vi "LNLS Control Encode FOFBC.vi"(8 "error in (no error)":errorcluster, 11 "LNLS Control FOFB Configuration":T1) -> (0 "error out":errorcluster, 2 "command body":string)   [LabVIEW 2011, in "LNLS Control VIs.lvlib"]
uses:
  LNLS Control VIs.lvlib
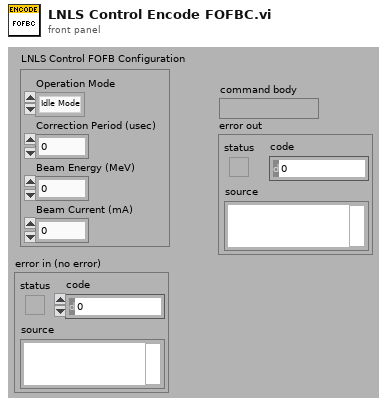
[diagram p1: front panel]
types:
  T1 = cluster{"Operation Mode":enum16{"Idle Mode", "Error Mode", "Manual Mode", "FOFB Mode", "RMM Mode"}, "Correction Period (usec)":i32, "Beam Energy (MeV)":sgl, "Beam Current (mA)":sgl}
  T2 = enum16{"big-endian, network order", "native, host order", "little-endian"}
  T3 = enum16{"Idle Mode", "Error Mode", "Manual Mode", "FOFB Mode", "RMM Mode"}
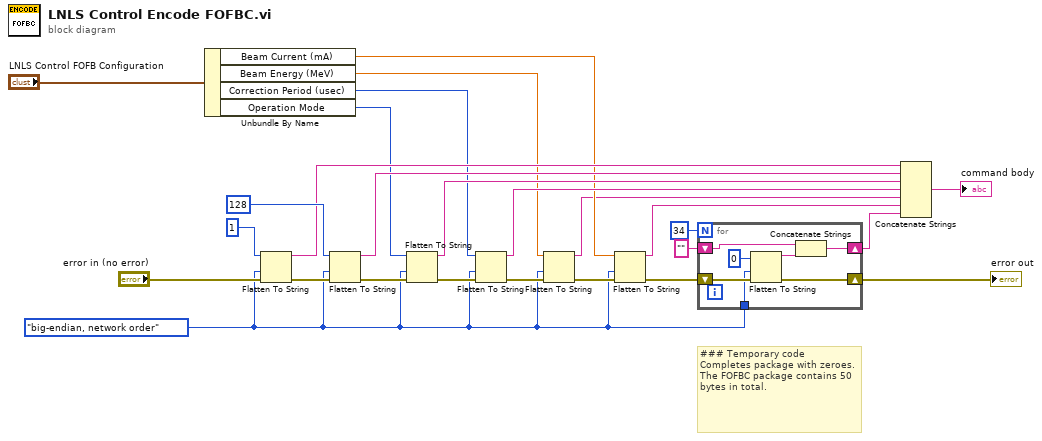
[diagram p0: block diagram]
diagram:
  w3 = T2."big-endian, network order" ("byte order (0:big-endian, network order)")
  # "### Temporary code\nCompletes package with zeroes. The FOFBC package contains 50 bytes in total."
  n1 = Unbundle By Name("LNLS Control FOFB Configuration") -> ("Beam Current (mA)"=w6:sgl, "Beam Energy (MeV)"=w7:sgl, "Correction Period (usec)"=w2:i32, "Operation Mode"=w1:T3)
  n2 = Flatten To String(anything=u8 1 ("Correction Period (usec)"), byte order (0:big-endian, network order)=w3, error in (no error)="error in (no error)") -> (data string=w17:string, error out=w19:errorcluster)  [unwired: 1 in, 1 out]
  n3 = Flatten To String(anything=u8 128 ("Correction Period (usec)"), byte order (0:big-endian, network order)=w3, error in (no error)=w19) -> (data string=w18:string, error out=w12:errorcluster)  [unwired: 1 in, 1 out]
  n4 = Flatten To String(anything=w1, byte order (0:big-endian, network order)=w3, error in (no error)=w12) -> (data string=w9:string, error out=w25:errorcluster)  [unwired: 1 in, 1 out]
  n5 = Flatten To String(anything=w2, byte order (0:big-endian, network order)=w3, error in (no error)=w25) -> (data string=w8:string, error out=w11:errorcluster)  [unwired: 1 in, 1 out]
  n6 = Flatten To String(anything=w7, byte order (0:big-endian, network order)=w3, error in (no error)=w11) -> (data string=w5:string, error out=w23:errorcluster)  [unwired: 1 in, 1 out]
  n7 = Flatten To String(anything=w6, byte order (0:big-endian, network order)=w3, error in (no error)=w23) -> (data string=w4:string, error out=w10:errorcluster)  [unwired: 1 in, 1 out]
  n8 = for {
    N: 34 -> [_]
    shift-right: [w32] -> w16
    shift-left: w10 -> [w33]
    shift-right: [w30] -> w14
    shift-left: "" -> [w29]
    tunnel: w3 -> [w27]
    n9 = Flatten To String(anything=u8 0 ("Correction Period (usec)"), byte order (0:big-endian, network order)=w27, error in (no error)=w33) -> (data string=w31:string, error out=w32:errorcluster)  [unwired: 1 in, 1 out]
    n10 = Concatenate Strings(w29, w31) -> (w30:string)
  }
  "error out" <- w16
  n11 = Concatenate Strings(w17, w18, w9, w8, w5, w4, w14) -> (→"command body":string)
